vi "Query Input.vi"(8 "error in":errorcluster, 11 "SL_SC in":refnum<class "SL_SC.lvclass">) -> (0 "error out":errorcluster, 1 "Input":u8[](array[numeric]), 3 "SL_SC out":refnum<class "SL_SC.lvclass">)   [LabVIEW 2019, in "SL_SC.lvlib" / "SL_SC.lvclass"]
doc: "This method must be overridden by the child class.\n\nThis should read the status at the input of the device and return a weform capture of the named signal states."
uses:
  Library/SL_SC.lvclass
  Library/SL_SC.lvclass/SL_SC.ctl
  <vilib>/SLSC/Get Generic Property (U32).vi
  <vilib>/SLSC/SLSC.lvlib
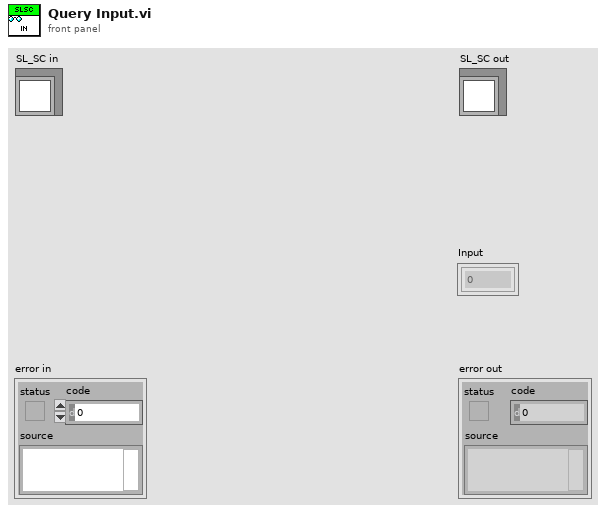
[diagram p1: front panel]
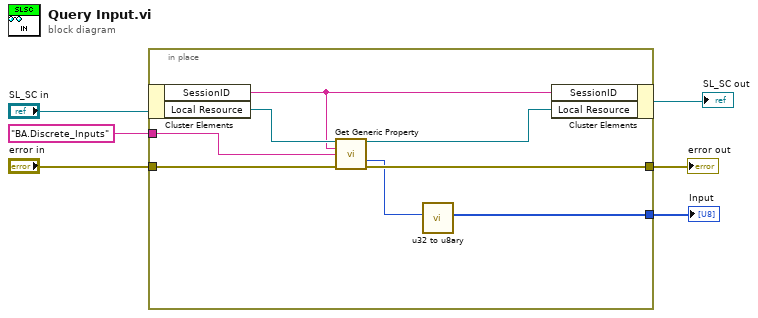
[diagram p0: block diagram]
diagram:
  n1 = in-place {
    in-place-border: [w12] -> w2
    in-place-border: "error in" -> [w11]
    in-place-border: [w10] -> w4
    in-place-border: "BA.Discrete_Inputs" -> [w9]
    n2 = in-place-cluster #1("SL_SC in") -> ("SessionID"=w8:string, "Local Resource"=w14:refnum<k21>)
    n3 = call-poly <vilib>:"Get Generic Property.vi"("session in"=w14, "resources"=w8, "property"=w9, "error in (no error)"=w11) -> ("session out"=w13:refnum<k21>, "property value"=w7:u32, "error out"=w10:errorcluster)  [unwired: 9 in]
    n4 = call "u32 to u8ary.vi"("Numeric"=w7) -> ("Array"=w12:u8[])  [unwired: 10 in]
    n5 = in-place-cluster #1("SessionID"=w8, "Local Resource"=w13) -> (→"SL_SC out":refnum<class "SL_SC.lvclass">)
  }
  "error out" <- w4
  "Input" <- w2
